vi "Get Name.vi"(8 "error in (no error)":errorcluster, 11 "SMO":refnum<class "SMO.lvclass">) -> (0 "error out":errorcluster, 1 "Given Name":string, 2 "Name":string, 3 "SMO out":refnum<class "SMO.lvclass">, 4 "Prospective Owner":string)   [LabVIEW 2021, in "smo.lvlib" / "SMO.lvclass"]
uses:
  SMO.lvclass
  Support/Attribute.Identity/Attribute.Identity.lvclass
  SMO.lvclass/SMO.ctl
  Support/Attribute.Identity/Attribute.Identity.lvclass/Attribute.Identity.ctl
  Private/ReftoDVR--SMO.vi
panel:
  # "This method is deprecated but kept for\nbackward-compatibility.\nUse the \"GetName.vi\" method instead of \"Get Name.vi\""
  # "For instructions on how to use the JKI State Machine Objects, examples and video tutorials, visit:\nhttp://jki.net/state-machine-objects/\n\nJKI State Machine Objects™\nhttp://jki.net/state-machine-objects/\nCopyright (C) 2005-2015, JKI <info@jki.net>\nALL RIGHTS RESERVED"
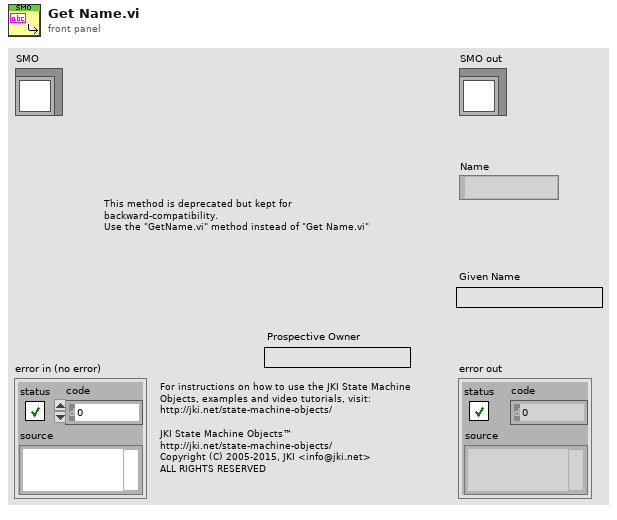
[diagram p1: front panel]
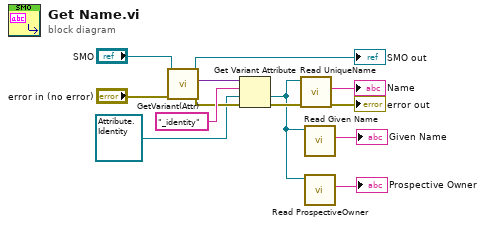
[diagram p0: block diagram]
diagram:
  n1 = call "GetVariant(Attr).vi"("error in (no error)"="error in (no error)", "SMO in"="SMO") -> ("error out"=w10:errorcluster, "[Attributes]"=w12:variant, "SMO out"=→"SMO out":refnum<class "SMO.lvclass">)  [unwired: 7 in]
  n2 = Get Variant Attribute(Variant=w12, name="_identity", default value (empty Variant)=refnum<class "Attribute.Identity.lvclass"> refnum, error in=w10) -> (value=w2:refnum<class "Attribute.Identity.lvclass">, error out=→"error out":errorcluster)  [unwired: 2 out]
  n3 = call "Read UniqueName.vi"("Attribute.Identity in"=w2) -> ("Unique Name"=→"Name":string)  [unwired: 9 in, 1 out]
  n4 = call "Read Given Name.vi"("Attribute.Identity in"=w2) -> ("Given Name"=→"Given Name":string)  [unwired: 9 in, 1 out]
  n5 = call "Read ProspectiveOwner.vi"("Attribute.Identity in"=w2) -> ("Prospective Owner"=→"Prospective Owner":string)  [unwired: 9 in, 1 out]
